vi "unstuff_bytes.vi"(11 "StuffedByteArrayIn":u8[](array[numeric])=[17, 19] format="%x") -> (3 "UnstuffedDataOut":u8[](array[numeric])=[17, 19] format="%x")   [LabVIEW 2019]
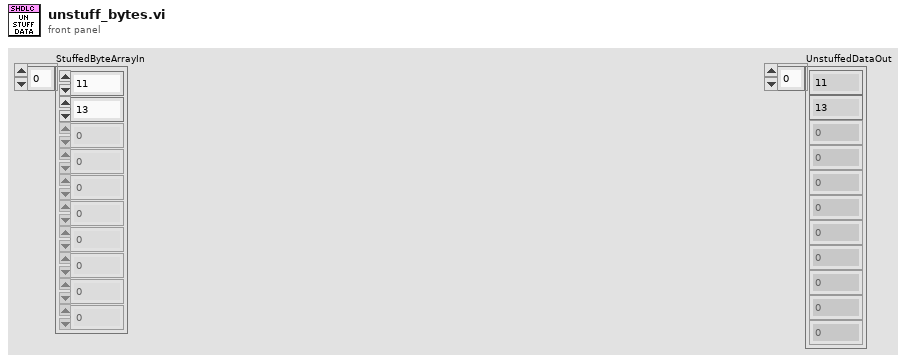
[diagram p1: front panel]
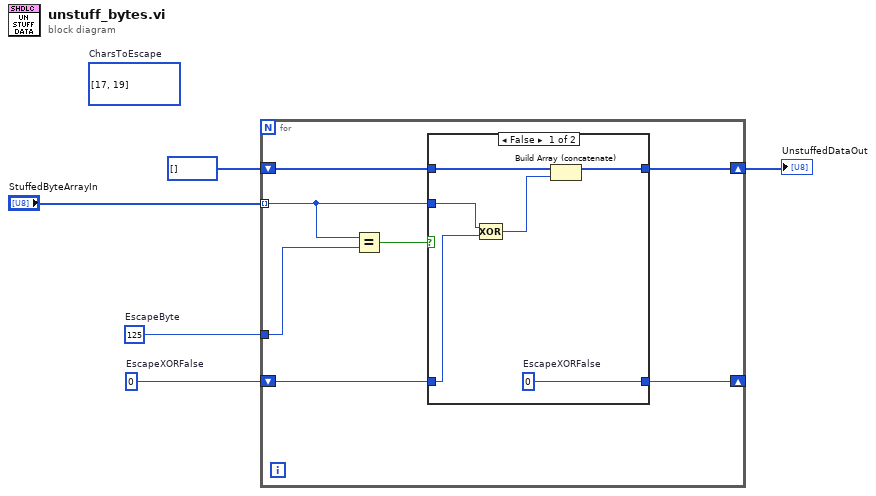
[diagram p0: block diagram]
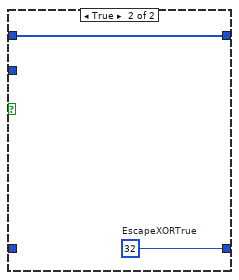
[diagram p2: hidden frame]
diagram:
  (unwired) u8[] [17, 19]  # CharsToEscape
  w2 = u8 0  # EscapeXORFalse
  w3 = u8 125  # EscapeByte
  n1 = for {
    tunnel: "StuffedByteArrayIn" -> [w11] mode=indexing
    shift-right: [w10] -> w1
    shift-left: u8[] [] ("ByteArrayIn 2") -> [w12]
    tunnel: w3 -> [w8]
    shift-right: [w6] -> _
    shift-left: w2 -> [w9]
    n2 = Equal?(x=w11, y=w8) -> (x = y?=w7:bool)
    n3 = case shown="False" w7 {
      tunnel: w12 -> [w18 w19]
      tunnel: w11 -> [w14 _]
      tunnel: [w17 w19] -> w10
      tunnel: w9 -> [w16 _]
      tunnel: [w13 w20] -> w6
      frame False {
        w13 = u8 0  # EscapeXORFalse
        n4 = Compound Arithmetic op=XOR(w14, w16) -> (w15:u8)
        n5 = Build Array (concatenate)(w18, w15) -> (w17:u8[])
      }
      frame True {
        w20 = u8 32  # EscapeXORTrue
      }
    }
  }
  "UnstuffedDataOut" <- w1
